vi "Begin.vi"(8 "error in":errorcluster) -> (0 "error out":errorcluster)   [LabVIEW 2018]
doc: "Called before other user functions, this VI is expected to open initial I/O refnums, load in file data, and do all program initialization. Notice that the <B>error out</B> terminal is simply used for data flow. Wiring it to other structures or subVIs ensures that this VI runs first."
uses:
  <vilib>/Rock Robotics/WPI/DriverStation/WPI_DriverStationRobotMode2.ctl
  <vilib>/Rock Robotics/WPI/Joystick/WPI_JoystickDeviceEnum.ctl
  Robot Global Data.vi
  <vilib>/Rock Robotics/Network Tables/NT Write String Array.vi
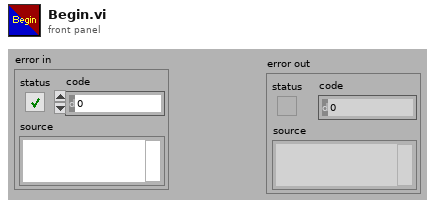
[diagram p1: front panel]
types:
  T1 = enum16{"FollowerType_PercentOutput", "FollowerType_AuxOutput1"}
  T2 = typedef "WPI_JoystickDeviceEnum.ctl" = enum16{"USB 0", "USB 1", "USB 2", "USB 3", "USB 4", "USB 5"}
  T3 = typedef "WPI_DriverStationRobotMode2.ctl" = enum16{"Autonomous Disabled", "Autonomous Enabled", "Teleop Disabled", "Teleop Enabled", "Disconnected", "Finish", "Test Disabled", "Test Enabled", "Emergency Stopped"}
  T4 = typedef "WPI_MotorControlDeviceRef.ctl" = cluster{"DeviceStatus":errorcluster, "Type":T5, "PWM":cluster{"PWM Channel":T6, "DeadBand":T7}, "CAN":cluster{"Device Number":u8, "SetOutput VI Ref":variant, "GetOutput VI Ref":variant, "Enable VI Ref":variant, "Disable VI Ref":variant, "Data":variant}, "Invert":bool, "DIO PWM":cluster{"PWM \"Enable\" Channel":T6, "DIOChannel":T8, "PWM Rate":dbl}}
  T5 = typedef "WPI_MotorControlType.ctl" = enum16{"PWM", "CAN", "DIO PWM"}
  T6 = typedef "FPGA_DIOPWMChannel.ctl" = enum8{"PWM 0", "PWM 1", "PWM 2", "PWM 3", "PWM 4", "PWM 5", "PWM 6", "PWM 7", "PWM 8", "PWM 9", "PWM MXP 0", "PWM MXP 1", "PWM MXP 2", "PWM MXP 3", "PWM MXP 4", "PWM MXP 5", "PWM MXP 6", "PWM MXP 7", "PWM MXP 8", "PWM MXP 9", "Invalid"}
  T7 = typedef "WPI_PWMDeadband.ctl" = cluster{"Name":string, "maxPositivePwm":i32, "minPositivePwm":i32, "centerPwm":i32, "maxNegativePwm":i32, "minNegativePwm":i32, "angularRange":u16}
  T8 = typedef "FPGA_DIOChannel.ctl" = enum8{"DIO 0", "DIO 1", "DIO 2", "DIO 3", "DIO 4", "DIO 5", "DIO 6", "DIO 7", "DIO 8", "DIO 9", "DIO MXP 0", "DIO MXP 1", "DIO MXP 2", "DIO MXP 3", "DIO MXP 4", "DIO MXP 5", "DIO MXP 6", "DIO MXP 7", "DIO MXP 8", "DIO MXP 9", "DIO MXP 10", "DIO MXP 11", "DIO MXP 12", "DIO MXP 13", "DIO MXP 14", "DIO MXP 15", "SPI Port CS1", "SPI Port CS2", "SPI Port CS3", "SPI Port MISO", "SPI Port MOSI", "Invalid"}
  T9 = typedef "WPI_JoystickDevRef.ctl" = cluster{"Device":T2}
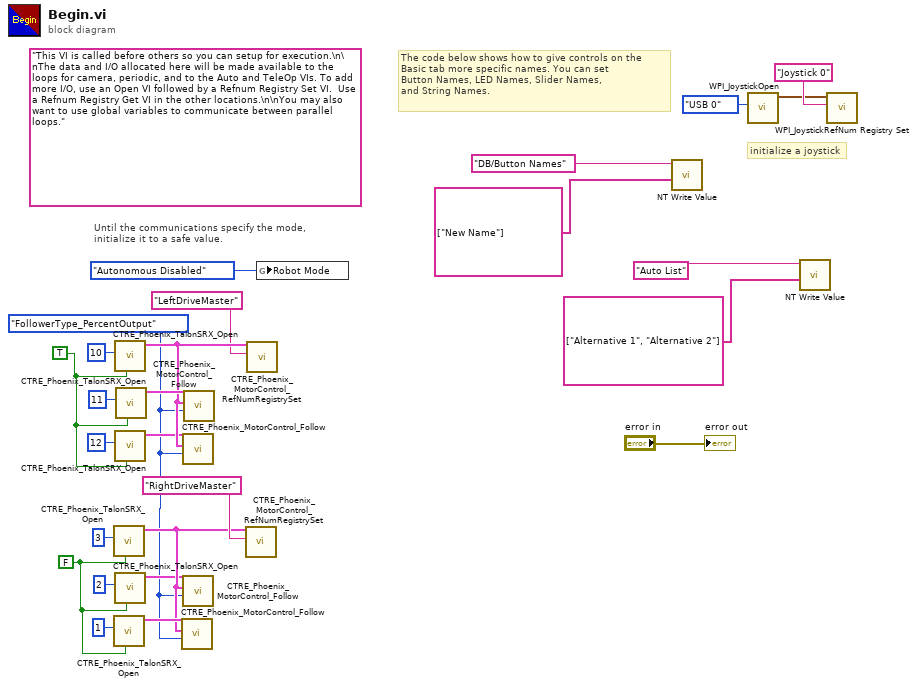
[diagram p0: block diagram]
diagram:
  w1 = TRUE ("Invert")
  w2 = FALSE ("Invert")
  w3 = T1."FollowerType_PercentOutput" ("FollowerType")
  (unwired) "This VI is called before others so you can setup for execution.\n\nThe data and I/O allocated here will be made available to the loops for camera, periodic, and to the Auto and TeleOp VIs. To add more I/O, use an Open VI followed by a Refnum Registry Set VI.  Use a Refnum Registry Get VI in the other locations.\n\nYou may also want to use global variables to communicate between parallel loops."
  # "The code below shows how to give controls on the\nBasic tab more specific names. You can set\nButton Names, LED Names, Slider Names,\nand String Names."
  # "initialize a joystick"
  # "Until the communications specify the mode,\ninitialize it to a safe value."
  n1 = call <vilib>:"CTRE_Phoenix_TalonSRX_Open.vi"("Invert"=w2, "Device Number"=u8 3) -> ("CAN Talon SRX Ref"=w8:T4)  [unwired: 8 in, 1 out]
  n2 = call <vilib>:"CTRE_Phoenix_TalonSRX_Open.vi"("Invert"=w2, "Device Number"=u8 1) -> ("CAN Talon SRX Ref"=w9:T4)  [unwired: 8 in, 1 out]
  n3 = call <vilib>:"CTRE_Phoenix_TalonSRX_Open.vi"("Invert"=w1, "Device Number"=u8 10) -> ("CAN Talon SRX Ref"=w13:T4)  [unwired: 8 in, 1 out]
  n4 = call <vilib>:"CTRE_Phoenix_TalonSRX_Open.vi"("Invert"=w1, "Device Number"=u8 12) -> ("CAN Talon SRX Ref"=w12:T4)  [unwired: 8 in, 1 out]
  n5 = call <vilib>:"CTRE_Phoenix_TalonSRX_Open.vi"("Invert"=w2, "Device Number"=u8 2) -> ("CAN Talon SRX Ref"=w6:T4)  [unwired: 8 in, 1 out]
  n6 = call <vilib>:"CTRE_Phoenix_TalonSRX_Open.vi"("Invert"=w1, "Device Number"=u8 11) -> ("CAN Talon SRX Ref"=w15:T4)  [unwired: 8 in, 1 out]
  n7 = call <vilib>:"CTRE_Phoenix_MotorControl_Follow.vi"("FollowerType"=w3, "Master Controller to Follow"=w8, "PhoenixMotorControlDevRef"=w9) -> ()  [unwired: 7 in, 2 out]
  n8 = call <vilib>:"CTRE_Phoenix_MotorControl_Follow.vi"("FollowerType"=w3, "Master Controller to Follow"=w13, "PhoenixMotorControlDevRef"=w12) -> ()  [unwired: 7 in, 2 out]
  n9 = call <vilib>:"CTRE_Phoenix_MotorControl_Follow.vi"("FollowerType"=w3, "Master Controller to Follow"=w8, "PhoenixMotorControlDevRef"=w6) -> ()  [unwired: 7 in, 2 out]
  n10 = call <vilib>:"CTRE_Phoenix_MotorControl_Follow.vi"("FollowerType"=w3, "Master Controller to Follow"=w13, "PhoenixMotorControlDevRef"=w15) -> ()  [unwired: 7 in, 2 out]
  n11 = call <vilib>:"CTRE_Phoenix_MotorControl_RefNumRegistrySet.vi"("refnum name"="RightDriveMaster", "PhoenixMotorControlDevRef"=w8) -> ()  [unwired: 8 in, 2 out]
  n12 = call <vilib>:"CTRE_Phoenix_MotorControl_RefNumRegistrySet.vi"("refnum name"="LeftDriveMaster", "PhoenixMotorControlDevRef"=w13) -> ()  [unwired: 8 in, 2 out]
  n13 = global write "Robot Global Data.vi" "Robot Mode"(WPI_DriverStationRobotMode2."Autonomous Disabled" ("Robot Mode")) -> ()
  n14 = call-poly <vilib>:"NT Write Value.vi"("String Array"=string[] ["New Name"], "Name"="DB/Button Names") -> ()  [unwired: 9 in, 1 out]
  n15 = call <vilib>:"WPI_JoystickOpen.vi"("JoystickDevice"=WPI_JoystickDeviceEnum."USB 0") -> ("JoystickDevRef"=w24:T9)  [unwired: 10 in]
  n16 = call-poly <vilib>:"NT Write Value.vi"("String Array"=string[] ["Alternative 1", "Alternative 2"], "Name"="Auto List") -> ()  [unwired: 9 in, 1 out]
  n17 = call <vilib>:"WPI_JoystickRefNum Registry Set.vi"("refnum name"="Joystick 0", "JoystickDevRef"=w24) -> ()  [unwired: 8 in, 2 out]
  "error out" <- "error in"
